vi "Module ID.vi"(11 "Redlines Module in":refnum<class "Redlines Module.lvclass">) -> (2 "Module ID":string)   [LabVIEW 2020, in "VolatusData.lvlib" / "Redlines Module.lvclass"]
uses:
  Redlines Module.lvclass
  Redlines Module.lvclass/Redlines Module.ctl
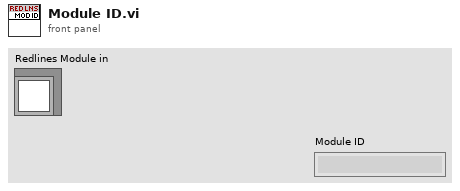
[diagram p1: front panel]
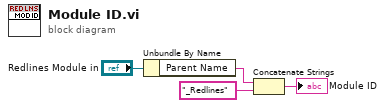
[diagram p0: block diagram]
diagram:
  n1 = Unbundle By Name("Redlines Module in") -> ("Parent Name"=w2:string)
  n2 = Concatenate Strings(w2, "_Redlines" ("string")) -> (→"Module ID":string)
